vi "Cam X.vi"() -> ()   [LabVIEW 2016]
panel:
  in  "Cam X":dbl
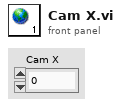
[diagram p1: front panel]
diagram:
